vi "simulator.vi"() -> ()   [LabVIEW 2010]
uses:
  TCL-Target_Computer_Logging/TCL Global.vi
  TCL-Target_Computer_Logging/TCL Select Fragments/TCL Select Fragments 1frag1criterium.vi
  TCL-Target_Computer_Logging/TCL Get Fragments/TCL Get Fragments - 1eventNfrag.vi
panel:
  in  "active baseline file":path
  in  "signal":string
  in  "simulate QCA signal":bool
  in  "period (s)":dbl
  in  "initiate events":bool
  in  "stop":bool
  out "next time to simulate":timestamp
  out "next event to simulate":u64
  out "last time processed":timestamp
  out "last time simulated":timestamp
  out "last event processed":u64
  out "last event simulated":u64
  in  "reset map":bool
  in  "first time to simulate":timestamp
  in  "first event to simulate":u64
  in  "primary key":string
  in  "simulation file":path
  in  "modules":T1(array[cluster])
  # "This VI allows one to simulate inputs from various PDP modules. When the enabled modules receive a GenEvent= message, they send the specified fragments to the Target Event Builder (TEB). The VI can send manually entered values for these fragments or read them sequentially from a simulus file, which should have the same format as an event file (one can simulate previous runs by loading in old event files).\n\nTo use this simulator:\n\n1. Configure the modules you want to simulate at right.\n2. In value mode, enter fragment names and their corresponding simulated values. In file mode, enter fragment names and their corresponding field names for file lookup. Repeat for each module.\n3. If using file mode, choose your data file (same format as event files) and select the first event number to simulate. By default, simulation will start with the first event in the file.\n4. Run PDP. Modules will respond to GenEvent= messages with the listed fragments.\n\nTo initiate TEB events periodically (a job that QCA normally handles), use the controls above. To simulate QCA signals, use the controls at top right."
  # "value"
  # "file"
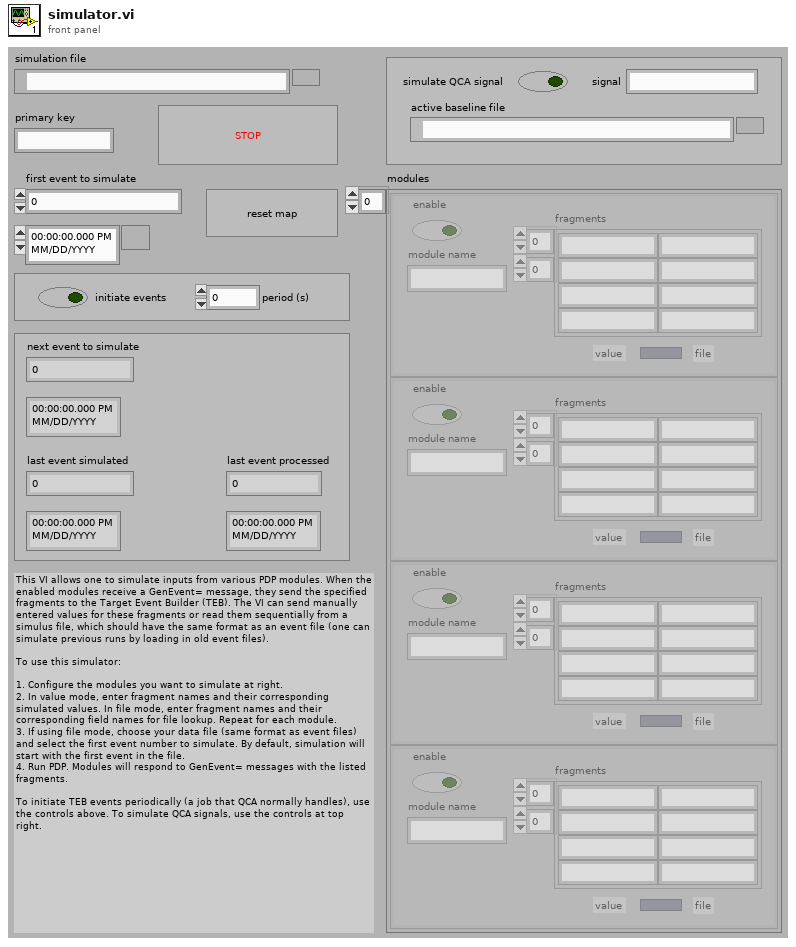
[diagram p1: front panel]
types:
  T1 = cluster{"enable":bool, "module name":string, "fragments":string[][], "file":bool}[]
  T2 = cluster{"fragment":string, "values":string[], "operator":string}
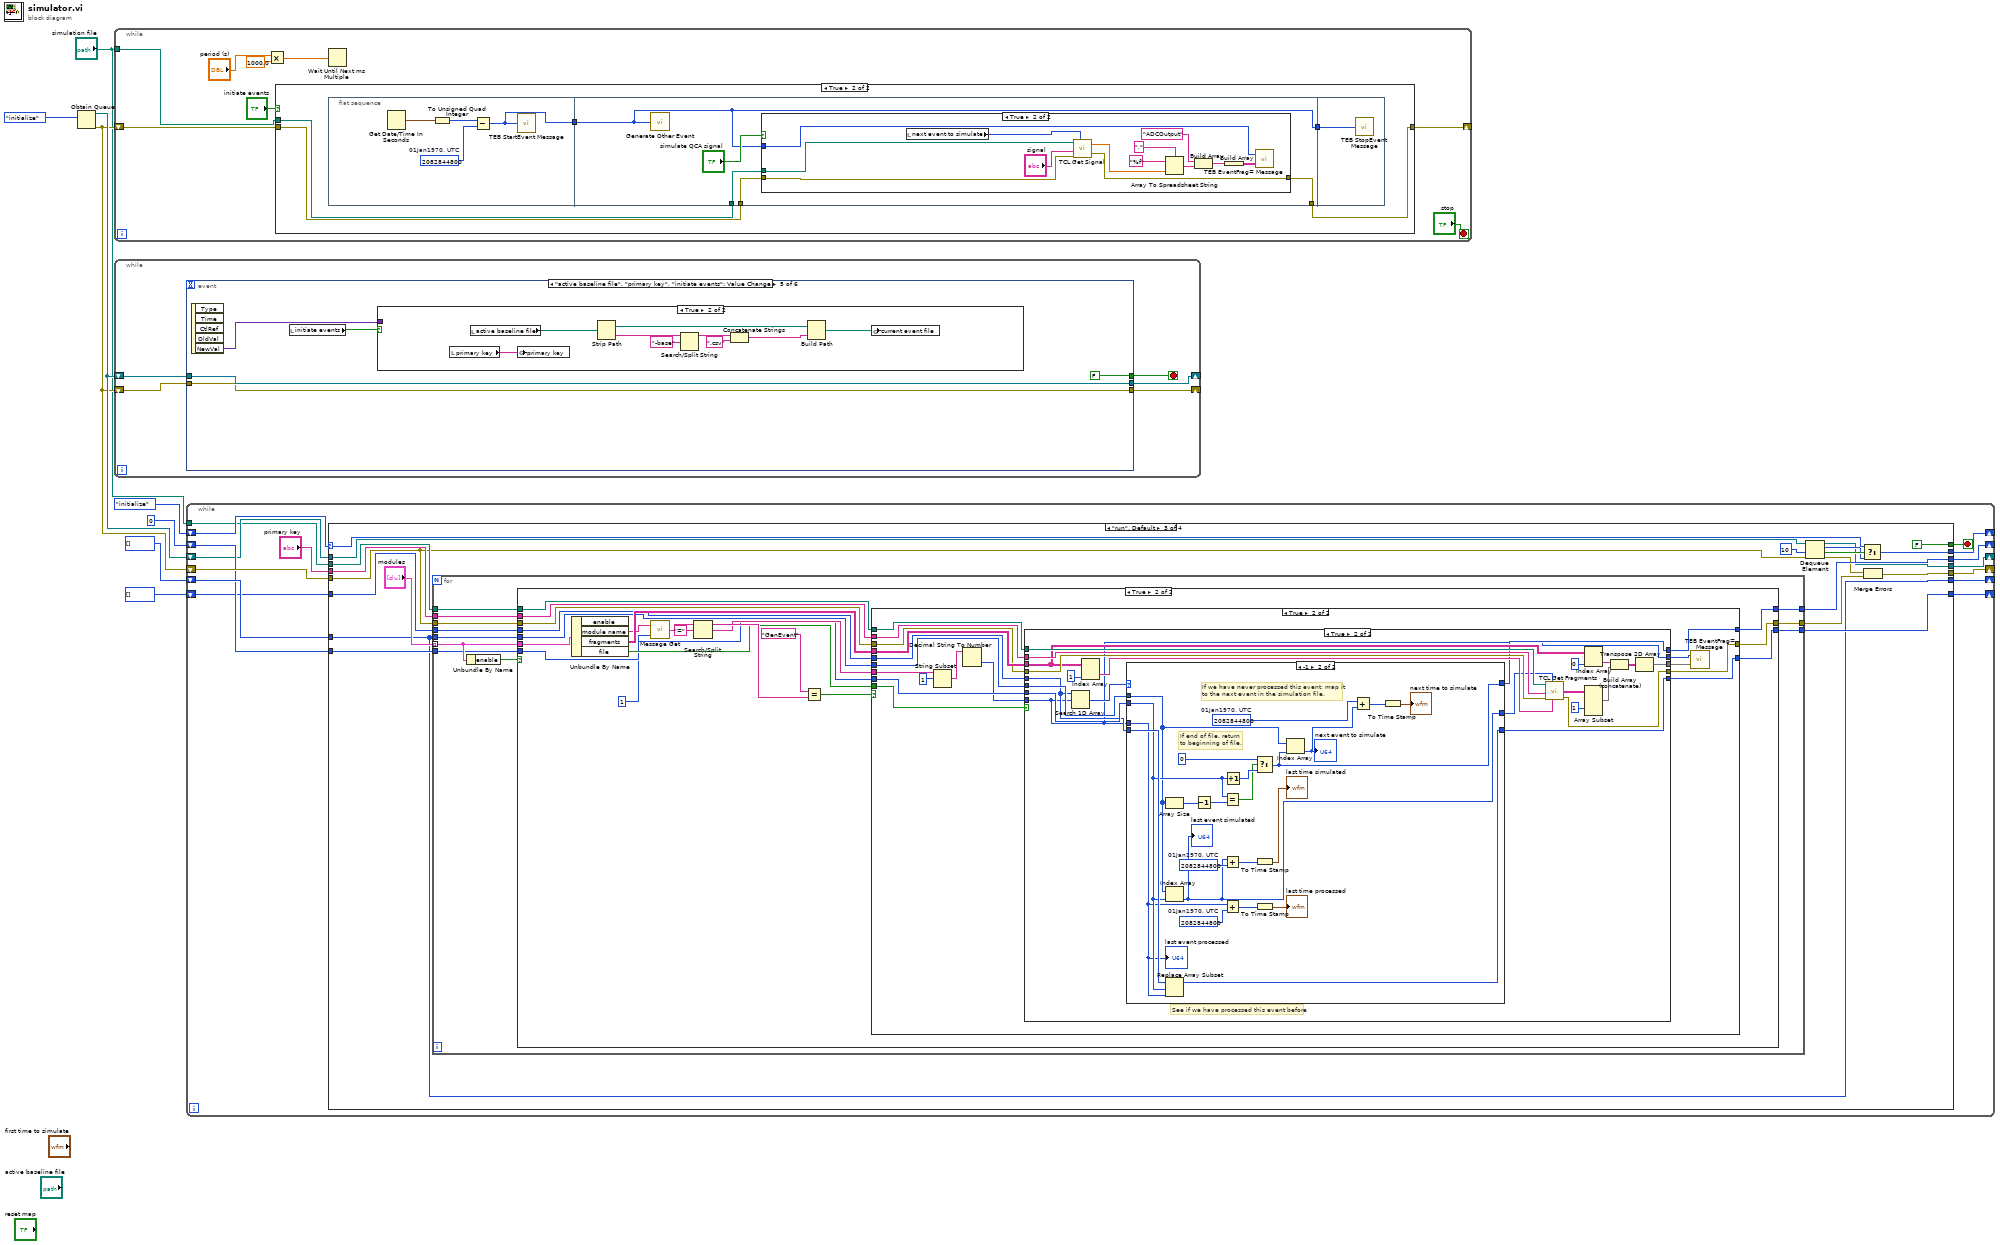
[diagram p0: block diagram]
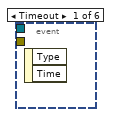
[diagram p4: hidden frame]
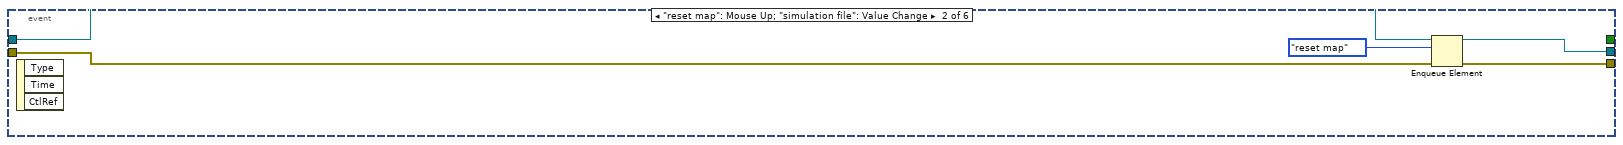
[diagram p5: hidden frame]
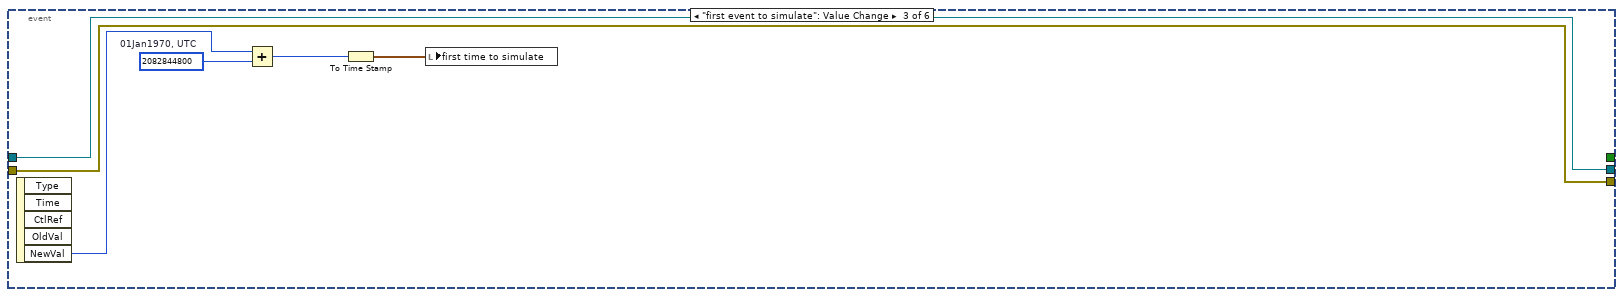
[diagram p6: hidden frame]
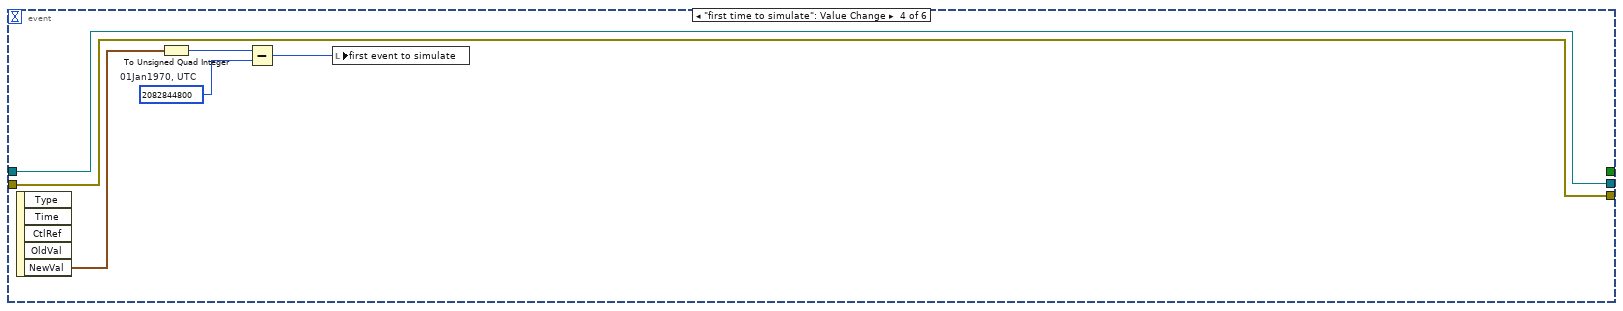
[diagram p7: hidden frame]
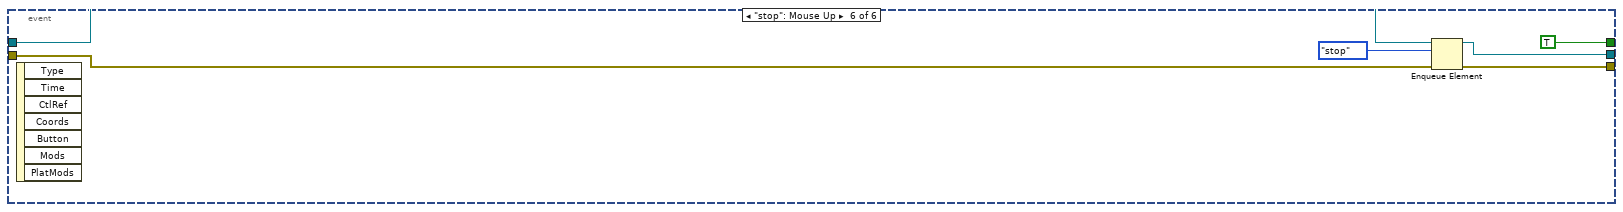
[diagram p9: hidden frame]
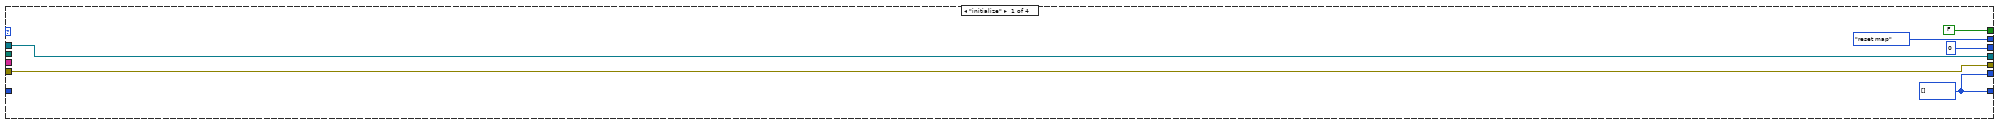
[diagram p10: hidden frame]
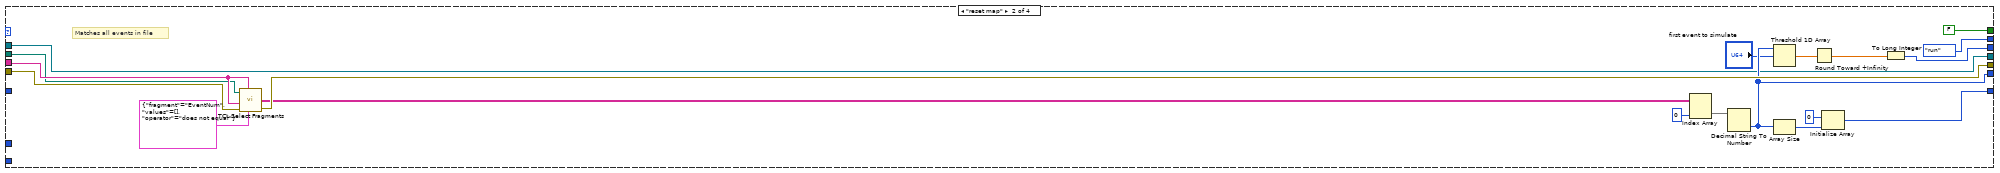
[diagram p11: hidden frame]
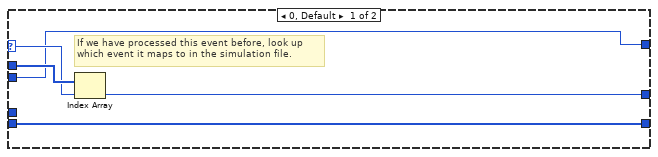
[diagram p15: hidden frame]
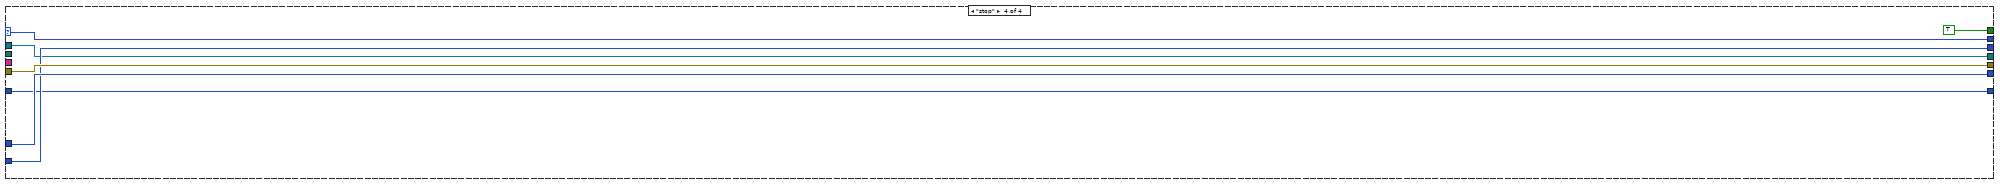
[diagram p16: hidden frame]
diagram:
  n1 = Obtain Queue(element data type=enum16{"initialize", "reset map", "run", "stop"}."initialize") -> (queue out=w3:refnum<queue>, error out=w2:errorcluster)  [unwired: 4 in, 1 out]
  n2 = while {
    tunnel: "simulation file" -> [w10]
    shift-right: [w9] -> _
    shift-left: w2 -> [w11]
    stop <- "stop" stop-if-true
    n3 = Multiply(x="period (s)", y=1000.0) -> (x*y=w13:dbl)
    n4 = case shown="True" "initiate events" {
      tunnel: w11 -> [w17 w20]
      tunnel: w10 -> [_ w19]
      tunnel: [w17 w18] -> w9
      frame False {
      }
      frame True {
        n5 = flat-sequence {
          tunnel: [w23] -> w22
          tunnel: w22 -> [w28]
          tunnel: [w28] -> w21
          tunnel: w20 -> [w30]
          tunnel: w19 -> [w29]
          tunnel: [w27] -> w18
          tunnel: w21 -> [w46]
          frame #0 {
            w25 = u64 2082844800  # 01Jan1970, UTC
            n6 = Get Date/Time In Seconds() -> (seconds since 1Jan1904=w26:timestamp)
            n7 = To Unsigned Quad Integer(1:w26) -> (0:w24:u64)
            n8 = Subtract(x=w24, y=w25) -> (x-y=w23:u64)
            n9 = call "TEB StartEvent Message.vi"("Event Number"=w23) -> ()
          }
          frame #1 {
            n10 = call "Generate Other Event.vi"("Event Number"=w28) -> ()
            n11 = case shown="True" "simulate QCA signal" {
              tunnel: w30 -> [w32 w44]
              tunnel: w29 -> [_ w43]
              tunnel: w28 -> [_ w41]
              tunnel: [w32 w42] -> w27
              frame False {
              }
              frame True {
                n12 = local read "next event to simulate"() -> (w33:u64)
                n13 = call "TCL Get Signal.vi"("event number"=w33, "error in (no error)"=w44, "signal name"="signal", "event file"=w43) -> ("error out"=w42:errorcluster, "signal"=w39:dbl[])  [unwired: 2 in]
                n14 = Array To Spreadsheet String(delimiter (Tab)=",", array=w39, 3:"%f" ("format string")) -> (spreadsheet string=w36:string)
                n15 = Build Array("ADCOutput", w36) -> (w35:string[])
                n16 = Build Array(w35) -> (w34:string[][])
                n17 = call "TEB EventFrag= Message.vi"("Event Fragment(s)"=w34, "Event Number"=w41) -> ()
              }
            }
          }
          frame #2 {
            n18 = call "TEB StopEvent Message.vi"("Event Number"=w46) -> ()
          }
        }
      }
    }
    n19 = Wait Until Next ms Multiple(millisecond multiple=w13) -> ()  [unwired: 1 out]
  }
  n20 = while {
    shift-right: [w48] -> _
    shift-left: w3 -> [w51]
    shift-right: [w49] -> _
    shift-left: w2 -> [w50]
    stop <- w47 stop-if-true
    n21 = event shown="[4] \"active baseline file\", \"primary key\", \"initiate events\": Value Change" {
      selector: _ -> [_ _ _ _ _ _]
      dyn-events: _ -> [_ _ _ _ _ _]
      timeout: _ -> [_ _ _ _ _ _]
      tunnel: w51 -> [_ w56 w58 w64 w71 w87]
      tunnel: w50 -> [_ w54 w57 w63 w70 w86]
      tunnel: [_ w53 w57 w63 w70 w85] -> w49
      tunnel: [_ w52 w58 w64 w71 w84] -> w48
      tunnel: [_ _ _ _ FALSE TRUE] -> w47
      event Timeout {
        n22 = event-data() -> ()  [unwired: 1 in, 2 out]
      }
      event "reset map": Mouse Up; "simulation file": Value Change {
        n23 = event-data() -> ()  [unwired: 1 in, 3 out]
        n24 = Enqueue Element(queue=w56, element=enum16{"initialize", "reset map", "run", "stop"}."reset map", error in (no error)=w54) -> (queue out=w52:refnum<queue>, error out=w53:errorcluster)  [unwired: 1 in, 1 out]
      }
      event "first event to simulate": Value Change {
        w61 = u64 2082844800  # 01Jan1970, UTC
        n25 = event-data() -> ("NewVal"=w62:u64)  [unwired: 1 in, 4 out]
        n26 = Add(x=w62, y=w61) -> (x+y=w60:u64)
        n27 = To Time Stamp(1:w60) -> (0:w59:timestamp)
        n28 = local write "first time to simulate"(w59) -> ()
      }
      event "first time to simulate": Value Change {
        w68 = u64 2082844800  # 01Jan1970, UTC
        n29 = event-data() -> ("NewVal"=w67:timestamp)  [unwired: 1 in, 4 out]
        n30 = To Unsigned Quad Integer(1:w67) -> (0:w65:u64)
        n31 = Subtract(x=w65, y=w68) -> (x-y=w66:u64)
        n32 = local write "first event to simulate"(w66) -> ()
      }
      event "active baseline file", "primary key", "initiate events": Value Change {
        n33 = event-data() -> ("NewVal"=w72:variant)  [unwired: 1 in, 4 out]
        n34 = local read "initiate events"() -> (w73:bool)
        n35 = case shown="True" w73 {
          tunnel: w72 -> [_ _]
          frame False {
          }
          frame True {
            n36 = local read "primary key"() -> (w82:string)
            n37 = local read "active baseline file"() -> (w81:path)
            n38 = global write "TCL Global.vi" "primary key"(w82) -> ()
            n39 = Strip Path(path=w81) -> (stripped path=w76:path, name=w80:string)
            n40 = Search/Split String(string=w80, search string/char (-)="-base") -> (substring before match=w78:string)  [unwired: 1 in, 2 out]
            n41 = Concatenate Strings(w78, ".csv" ("string")) -> (w75:string)
            n42 = Build Path(base path=w76, name or relative path=w75) -> (appended path=w74:path)
            n43 = global write "TCL Global.vi" "current event file"(w74) -> ()
          }
        }
      }
      event "stop": Mouse Up {
        n44 = event-data() -> ()  [unwired: 1 in, 7 out]
        n45 = Enqueue Element(queue=w87, element=enum16{"initialize", "reset map", "run", "stop"}."stop", error in (no error)=w86) -> (queue out=w84:refnum<queue>, error out=w85:errorcluster)  [unwired: 1 in, 1 out]
      }
    }
  }
  n46 = while {
    shift-right: [w100] -> _
    shift-left: enum16{"initialize", "reset map", "run", "stop"}."initialize" -> [w103]
    shift-right: [w99] -> _
    shift-left: w2 -> [w101]
    shift-right: [w97] -> _
    shift-left: i32[] [] -> [w98]
    shift-right: [w96] -> _
    shift-left: i32[] [] -> [w92]
    shift-right: [w95] -> _
    shift-left: 0 ("String") -> [w94]
    shift-right: [w91] -> _
    shift-left: w3 -> [w90]
    tunnel: "simulation file" -> [w89]
    stop <- w102 stop-if-true
    n47 = case shown="\"run\", Default" w103 {
      selector: w103 -> [_ _ w131 w263]
      tunnel: [FALSE FALSE FALSE TRUE] -> w102
      tunnel: w101 -> [w107 w126 w138 w262]
      tunnel: [enum16{"initialize", "reset map", "run", "stop"}."reset map" enum16{"initialize", "reset map", "run", "stop"}."run" w132 w263] -> w100
      tunnel: [w107 w125 w134 w262] -> w99
      tunnel: w98 -> [_ _ w140 w260]
      tunnel: [w106 w117 w140 w260] -> w97
      tunnel: [w106 w119 w141 w258] -> w96
      tunnel: [0 ("String") w113 w142 w259] -> w95
      tunnel: w94 -> [_ _ w144 w259]
      tunnel: "primary key" -> [_ w112 w146 _]
      tunnel: w89 -> [_ w111 w145 _]
      tunnel: w92 -> [_ _ w143 w258]
      tunnel: [w104 w110 w129 w257] -> w91
      tunnel: w90 -> [w104 w110 w139 w257]
      frame "initialize" {
        w106 = i32[] []
      }
      frame "reset map" {
        # "Matches all events in file"
        n48 = call-poly "TCL Select Fragments.vi"("event file"=w111, "fragment"=w112, "primary key"=w112, "criterium"=T2 {"fragment"="EventNum", "values"=[], "operator"="does not equal"}, "error in (no error)"=w126) -> ("matches"=w123:string[][], "error out"=w125:errorcluster)  [unwired: 1 in, 1 out]
        n49 = Index Array(array=w123, index (col)=0 ("disabled index (col)")) -> (element=w121:string[])  [unwired: 1 in]
        n50 = Decimal String To Number(string=w121) -> (number=w117:i32[])  [unwired: 2 in, 1 out]
        n51 = Threshold 1D Array(2:"first event to simulate", 3:w117) -> (0:w115:dbl)  [unwired: 1 in]
        n52 = Array Size(array=w117) -> (size(s)=w120:i32)
        n53 = Round Toward +Infinity(x=w115) -> (ceil(x): smallest int >= x=w114:dbl)
        n54 = Initialize Array(0 ("String"), w120) -> (w119:i32[])
        n55 = To Long Integer(number=w114) -> (32bit integer=w113:i32)
      }
      frame "run", Default {
        n56 = for {
          tunnel: "modules" -> [w158] mode=indexing
          tunnel: w140 -> [w157]
          tunnel: w144 -> [w156]
          tunnel: w138 -> [w155]
          tunnel: [w154] -> w135
          tunnel: w146 -> [w153]
          tunnel: w145 -> [w152]
          tunnel: w143 -> [w151]
          tunnel: [w150] -> w142
          tunnel: [w149] -> w141
          n57 = Unbundle By Name(w158) -> ("enable"=w159:bool)
          n58 = case shown="True" w159 {
            tunnel: w158 -> [_ w182]
            tunnel: w157 -> [_ w173]
            tunnel: w156 -> [w161 w172]
            tunnel: w155 -> [w162 w171]
            tunnel: [w162 w170] -> w154
            tunnel: w153 -> [_ w169]
            tunnel: w152 -> [_ w168]
            tunnel: w151 -> [w160 w167]
            tunnel: [w161 w166] -> w150
            tunnel: [w160 w165] -> w149
            frame False {
            }
            frame True {
              n59 = Unbundle By Name(w182) -> ("module name"=w164:string, "fragments"=w175:string[][], "file"=w174:bool)  [unwired: 1 out]
              n60 = call "Message Get.vi"("Timeout ms (-1)"=1, "Module"=w164) -> ("data out"=w179:string)
              n61 = Search/Split String(string=w179, search string/char (-)="=") -> (substring before match=w177:string, match + rest of string=w176:string)  [unwired: 1 in, 1 out]
              n62 = Equal?(x="GenEvent", y=w177) -> (x = y?=w180:bool)
              n63 = case shown="True" w180 {
                tunnel: w176 -> [_ w201]
                tunnel: w175 -> [_ w198]
                tunnel: w174 -> [_ w199]
                tunnel: w173 -> [_ w196]
                tunnel: w172 -> [w184 w195]
                tunnel: w171 -> [w185 w194]
                tunnel: [w185 w193] -> w170
                tunnel: w169 -> [_ w192]
                tunnel: w168 -> [_ w191]
                tunnel: w167 -> [w183 w190]
                tunnel: [w184 w189] -> w166
                tunnel: [w183 w188] -> w165
                frame False {
                }
                frame True {
                  n64 = String Subset(string=w201, offset (0)=1) -> (substring=w200:string)  [unwired: 1 in]
                  n65 = Decimal String To Number(string=w200) -> (number=w187:i32)  [unwired: 2 in, 1 out]
                  n66 = case shown="True" w199 {
                    tunnel: w198 -> [w207 w223]
                    tunnel: [w207 w218] -> w197
                    tunnel: w196 -> [_ w214]
                    tunnel: w195 -> [w205 w212]
                    tunnel: w194 -> [w206 w227]
                    tunnel: [w206 w226] -> w193
                    tunnel: w192 -> [_ w225]
                    tunnel: w191 -> [_ w224]
                    tunnel: w187 -> [w203 w208]
                    tunnel: w190 -> [w204 w210]
                    tunnel: [w205 w211] -> w189
                    tunnel: [w204 w209] -> w188
                    tunnel: [w203 w208] -> w186
                    frame False {
                    }
                    frame True {
                      # "See if we have processed this event before"
                      n67 = Search 1D Array(1D array=w210, element=w208) -> (index of element=w215:i32)  [unwired: 1 in]
                      n68 = Index Array(array=w223, index (col)=1 ("disabled index (col)")) -> (element=w228:string[])  [unwired: 1 in]
                      n69 = case shown="-1" w215 {
                        selector: w215 -> [w233 _]
                        tunnel: w214 -> [w234 w248]
                        tunnel: [w232 w241] -> w213
                        tunnel: w212 -> [w231 w251]
                        tunnel: [w231 w247] -> w211
                        tunnel: w210 -> [w230 w256]
                        tunnel: w208 -> [_ w246]
                        tunnel: [w230 w249] -> w209
                        frame 0, Default {
                          # "If we have processed this event before, look up\nwhich event it maps to in the simulation file."
                          n70 = Index Array(array=w234, index=w233) -> (element=w232:i32)
                        }
                        frame -1 {
                          w238 = u64 2082844800  # 01Jan1970, UTC
                          w242 = u64 2082844800  # 01Jan1970, UTC
                          w245 = u64 2082844800  # 01Jan1970, UTC
                          # "If end of file, return\nto beginning of file."
                          # "If we have never processed this event, map it\nto the next event in the simulation file."
                          n71 = Array Size(array=w248) -> (size(s)=w254:i32)
                          n72 = Index Array(array=w248, index=w251) -> (element=w241:i32)
                          "last event simulated" <- w241
                          n73 = Replace Array Subset(array=w256, new element=w246, index=w251) -> (w249:i32[])
                          n74 = Decrement(x=w254) -> (x-1=w252:i32)
                          n75 = Equal?(x=w251, y=w252) -> (x = y?=w250:bool)
                          n76 = Add(x=w241, y=w242) -> (x+y=w240:u64)
                          n77 = Add(x=w246, y=w245) -> (x+y=w244:u64)
                          n78 = Increment(x=w251) -> (x+1=w255:i32)
                          n79 = Select(t=0, s=w250, f=w255) -> (s? t:f=w247:i32)
                          n80 = To Time Stamp(1:w240) -> (0:→"last time simulated":timestamp)
                          n81 = To Time Stamp(1:w244) -> (0:→"last time processed":timestamp)
                          n82 = Index Array(array=w248, index=w247) -> (element=w237:i32)
                          "next event to simulate" <- w237
                          n83 = Add(x=w238, y=w237) -> (x+y=w236:u64)
                          n84 = To Time Stamp(1:w236) -> (0:→"next time to simulate":timestamp)
                          "last event processed" <- w246
                        }
                      }
                      n85 = call-poly "TCL Get Fragments.vi"("event file"=w224, "event number"=w213, "primary key"=w225, "fragments"=w228, "error in (no error)"=w227) -> ("values"=w220:string[][], "error out"=w226:errorcluster)  [unwired: 1 in, 1 out]
                      n86 = Index Array(array=w223, index (col)=0 ("disabled index (col)")) -> (element=w221:string[])  [unwired: 1 in]
                      n87 = Array Subset(array=w220, index (col)=1 ("index")) -> (w217:string[][])  [unwired: 3 in]
                      n88 = Build Array (concatenate)(w221, w217) -> (w219:string[][])
                      n89 = Transpose 2D Array(2D array=w219) -> (transposed array=w218:string[][])
                    }
                  }
                  n90 = call "TEB EventFrag= Message.vi"("Event Fragment(s)"=w197, "Event Number"=w186) -> ()
                }
              }
            }
          }
        }
        n91 = Dequeue Element(queue=w139, timeout in ms (-1)=10, error in (no error)=w138) -> (queue out=w129:refnum<queue>, element=w130:enum16{"initialize", "reset map", "run", "stop"}, timed out?=w133:bool, error out=w136:errorcluster)
        n92 = Select(t=w131, s=w133, f=w130) -> (s? t:f=w132:enum16{"initialize", "reset map", "run", "stop"})
        n93 = Merge Errors(w136, w135) -> (w134:errorcluster)
      }
      frame "stop" {
      }
    }
  }
